vi "Write to DSC.vi"(8 "error in (no error)":errorcluster, 9 "Variant":variant, 10 "Address":string, 11 "Logger in":refnum<class "Logger.lvclass">) -> (0 "error out":errorcluster, 3 "Logger out":refnum<class "Logger.lvclass">)   [LabVIEW 2016, in "Logger.lvclass"]
uses:
  Logger.lvclass
  C:/Program Files (x86)/National Instruments/LabVIEW 2016/vi.lib/JKI/JKI SMO/SMO/SMO.lvclass
  Logger.lvclass/Logger.ctl
  <vilib>/JKI/JKI SMO/URI Parsing/URI.lvlib
  <vilib>/JKI/JKI SMO/SMO/SMO.lvclass
  <vilib>/Utility/Data Type/NI_Data Type.lvlib
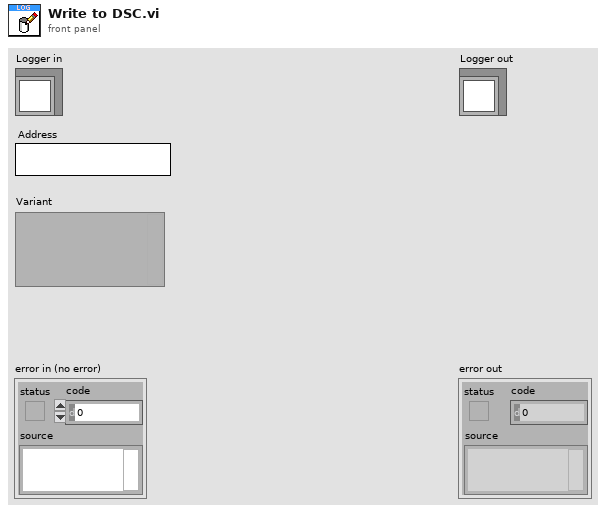
[diagram p1: front panel]
types:
  T1 = typedef "NI_Data Type.lvlib/Data Type.ctl" = enum8{"Invalid Type", "Void", "I8", "I16", "I32", "I64", "U8", "U16", "U32", "U64", "Single Float", "Double Float", "Extended Float", "Single Complex", "Double Complex", "Extended Complex", "Enum U8", "Enum U16", "Enum U32", "Enum U64", "Single Float With Unit", "Double Float With Unit", "Extended Float With Unit", "Single Complex with Unit", "Double Complex with Unit", "Extended Complex with Unit", "Boolean", "String", "Path", "Picture", "Tag", "Array", "Cluster", "Variant", "LV Variant", "Waveform", "Timestamp", "Digital Waveform", "Digital Data", "ExpressData", "Refnum", "External Data", "VI", "Poly VI", "LabVIEW Class Instance", "Fixed Point"}
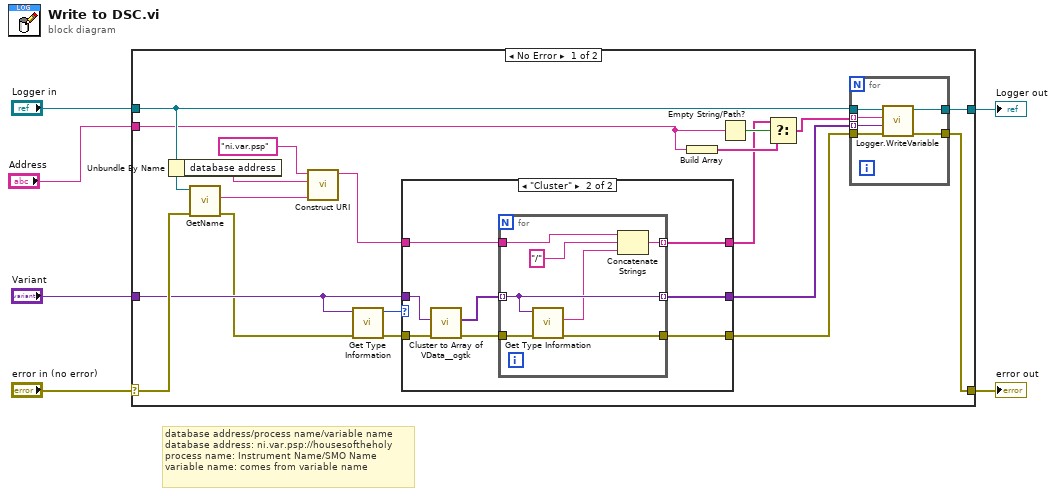
[diagram p0: block diagram]
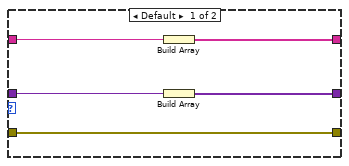
[diagram p2: hidden frame]
diagram:
  # "database address/process name/variable name\ndatabase address: ni.var.psp://housesoftheholy\nprocess name: Instrument Name/SMO Name\nvariable name: comes from variable name"
  n1 = case shown="No Error" "error in (no error)" {
    selector: "error in (no error)" -> [w12 w53]
    tunnel: [w21 w53] -> w5
    tunnel: [w25 w52] -> w3
    tunnel: "Logger in" -> [w19 w52]
    tunnel: "Variant" -> [w11 _]
    tunnel: "Address" -> [w9 _]
    frame No Error {
      n2 = Unbundle By Name(w19) -> ("database address"=w23:string)
      n3 = call <vilib>:"GetName.vi"("error in (no error)"=w12, "SMO"=w19) -> ("error out"=w10:errorcluster, "Name"=w20:string)  [unwired: 7 in, 1 out]
      n4 = call <vilib>:"Construct URI.vi"("path"=w20, "address"=w23, "protocol"="ni.var.psp") -> ("URI"=w7:string)  [unwired: 8 in]
      n5 = call <vilib>:"Get Type Information.vi"("error in (no error)"=w10, "Variant"=w11) -> ("error out"=w8:errorcluster, "Type"=w16:T1)  [unwired: 5 in, 3 out]
      n6 = case shown="\"Cluster\"" w16 {
        tunnel: w7 -> [w30 w37]
        tunnel: [w26 w36] -> w22
        tunnel: [w29 w35] -> w14
        tunnel: w11 -> [w28 w34]
        tunnel: [w27 w31] -> w15
        tunnel: w8 -> [w26 w32]
        frame Default {
          n7 = Build Array(w30) -> (w29:string[])
          n8 = Build Array(w28) -> (w27:variant[])
        }
        frame "Cluster" {
          n9 = call <userlib>:"Cluster to Array of VData__ogtk.vi"("error in (no error)"=w32, "Cluster"=w34) -> ("error out"=w38:errorcluster, "Array of VData"=w33:variant[])  [unwired: 8 in]
          n10 = for {
            tunnel: w33 -> [w42] mode=indexing
            tunnel: w38 -> [w45]
            tunnel: w37 -> [w40]
            tunnel: [w44] -> w35 mode=indexing
            tunnel: [w43] -> w36
            tunnel: [w42] -> w31 mode=indexing
            n11 = call <vilib>:"Get Type Information.vi"("error in (no error)"=w45, "Variant"=w42) -> ("error out"=w43:errorcluster, "Name"=w41:string)  [unwired: 5 in, 3 out]
            n12 = Concatenate Strings(w40, "/" ("string"), w41) -> (w44:string)
          }
        }
      }
      n13 = Build Array(w9) -> (w17:string[])
      n14 = Empty String/Path?(string/path=w9) -> (empty?=w18:bool)
      n15 = Select(t=w14, s=w18, f=w17) -> (s? t:f=w13:string[])
      n16 = for {
        tunnel: w19 -> [w50]
        tunnel: [w51] -> w25
        tunnel: w15 -> [w49] mode=indexing
        tunnel: w13 -> [w48] mode=indexing
        tunnel: w22 -> [w47]
        tunnel: [w46] -> w21
        n17 = call "Logger.WriteVariable.vi"("error in (no error)"=w47, "Data"=w49, "Address"=w48, "Logger"=w50) -> ("error out"=w46:errorcluster, "Logger out"=w51:refnum<class "Logger.lvclass">)  [unwired: 6 in]
      }
    }
    frame Error {
    }
  }
  "error out" <- w5
  "Logger out" <- w3
